vi "alpha_k.vi"(6 "u(t)":dbl[][](array[numeric]), 7 "alk":dbl[][](array[numeric]), 8 "nontarget_covariance":dbl[][](array[numeric]), 9 "target_covariance":dbl[][](array[numeric]), 11 "alpha(t-1)":ext[](array[numeric])) -> (3 "alpha(t)":ext[](array[numeric]))   [LabVIEW 2013]
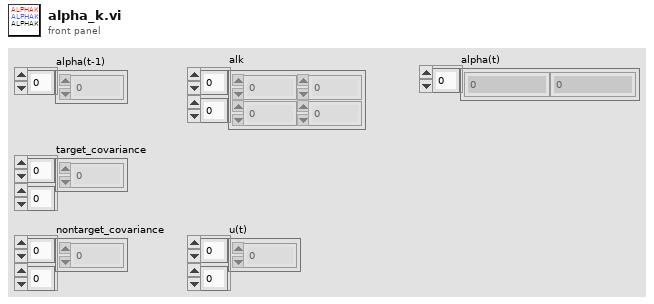
[diagram p1: front panel]
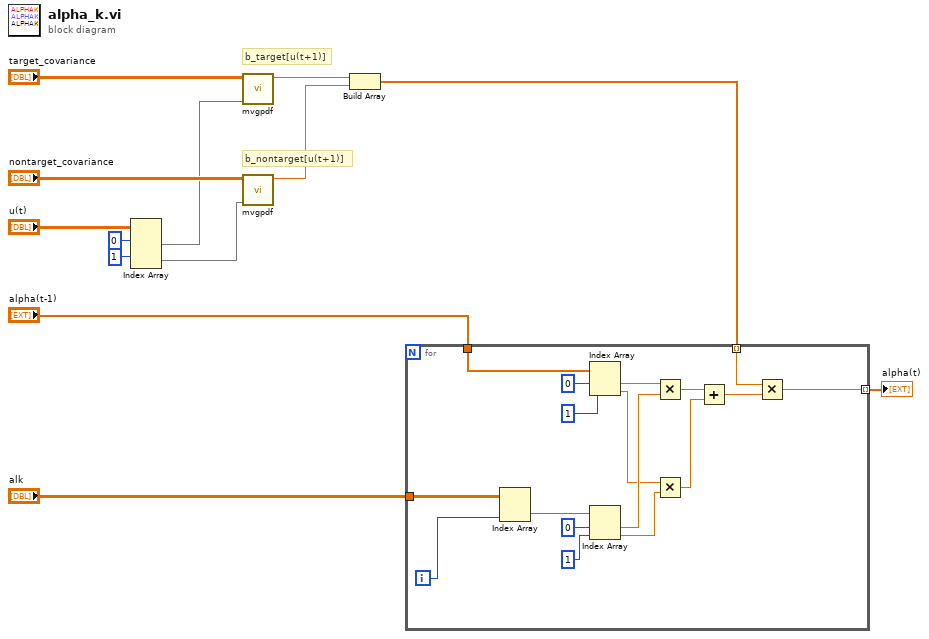
[diagram p0: block diagram]
diagram:
  # "b_nontarget[u(t+1)]"
  # "b_target[u(t+1)]"
  n1 = Index Array(array="u(t)", index (row) #1=0 ("index (row)"), index (row) #2=1 ("index (row)")) -> (element #1=w5:dbl[], element #2=w3:dbl[])  [unwired: 2 in]
  n2 = call "mvgpdf.vi"("input_ERP(normalized)"=w5, "covariance"="target_covariance") -> ("Gaussian_prob"=w9:ext)  [unwired: 9 in]
  n3 = call "mvgpdf.vi"("input_ERP(normalized)"=w3, "covariance"="nontarget_covariance") -> ("Gaussian_prob"=w8:ext)  [unwired: 9 in]
  n4 = Build Array(w9, w8) -> (w7:ext[])
  n5 = for {
    tunnel: "alk" -> [w27]
    tunnel: "alpha(t-1)" -> [w21]
    tunnel: w7 -> [w15] mode=indexing
    tunnel: [w14] -> w6 mode=indexing
    i -> [w26]
    n6 = Index Array(array=w27, index (col)=w26) -> (element=w28:dbl[])  [unwired: 1 in]
    n7 = Index Array(array=w21, index #1=0 ("index"), index #2=1 ("index")) -> (element #1=w18:ext, element #2=w17:ext)
    n8 = Index Array(array=w28, index #1=0 ("index"), index #2=1 ("index")) -> (element #1=w25:dbl, element #2=w24:dbl)
    n9 = Multiply(x=w18, y=w25) -> (x*y=w23:ext)
    n10 = Multiply(x=w17, y=w24) -> (x*y=w22:ext)
    n11 = Add(x=w23, y=w22) -> (x+y=w16:ext)
    n12 = Multiply(x=w15, y=w16) -> (x*y=w14:ext)
  }
  "alpha(t)" <- w6
